vi "mqttBuildClientID.vi"(0 "mqtt in":refnum<class "mqtt.lvclass">, 11 "error in (no error)":errorcluster) -> (4 "mqtt out":refnum<class "mqtt.lvclass">, 8 "clientID out":u8[](array[numeric]), 15 "error out":errorcluster)   [LabVIEW 2018, in "labview-mqtt.lvlib" / "mqtt.lvclass"]
uses:
  mqtt.lvclass
  mqtt.lvclass/mqtt.ctl
  labview-mqtt.lvlib
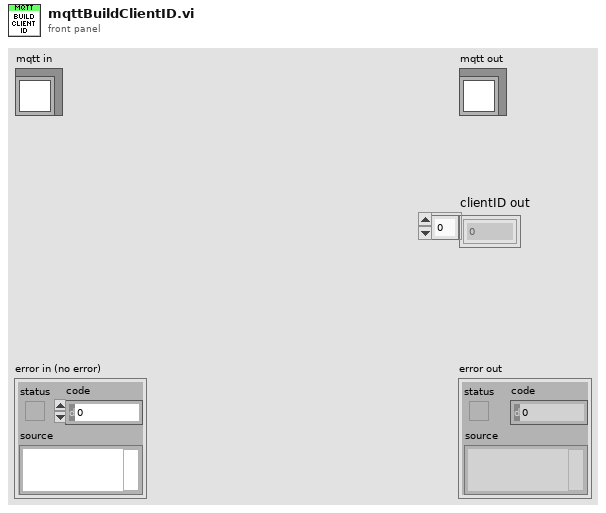
[diagram p1: front panel]
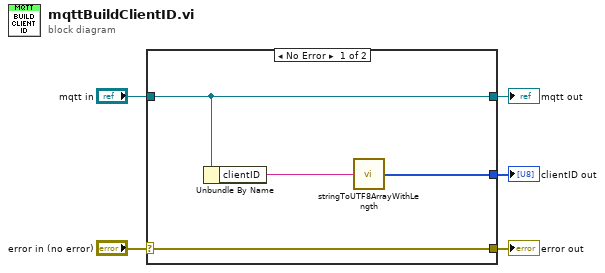
[diagram p0: block diagram]
diagram:
  n1 = case shown="No Error" "error in (no error)" {
    selector: "error in (no error)" -> [w9 w11]
    tunnel: [w9 w11] -> w4
    tunnel: [w8 w10] -> w2
    tunnel: "mqtt in" -> [w8 w10]
    tunnel: [w6 _] -> w1
    frame No Error {
      n2 = Unbundle By Name(w8) -> ("clientID"=w7:string)
      n3 = call "stringToUTF8ArrayWithLength.vi"("string"=w7) -> ("UTF8[]"=w6:u8[])  [unwired: 14 in]
    }
    frame Error {
    }
  }
  "error out" <- w4
  "mqtt out" <- w2
  "clientID out" <- w1
